vi "FrontPanelManager_Init.vi"(0 "reference in":refnum<class "FrontPanelManager.lvclass"> caption="This control should only be used when\na sub class is inheriting this class", 2 "Websocket Info":T1, 5 "error in (no error)":errorcluster) -> (14 "reference out":refnum<class "FrontPanelManager.lvclass"> caption="This indicator should only be used when\na sub class is inheriting this class", 19 "error out":errorcluster)   [LabVIEW 2014, in "FrontPanelPublisher.lvlib" / "FrontPanelManager.lvclass"]
uses:
  FrontPanelManager.lvclass
  Controls/WebsocketInfo.ctl
  WebFrontPanel_class/WebFrontPanel.lvclass
  Websocket_class/Websocket.lvclass
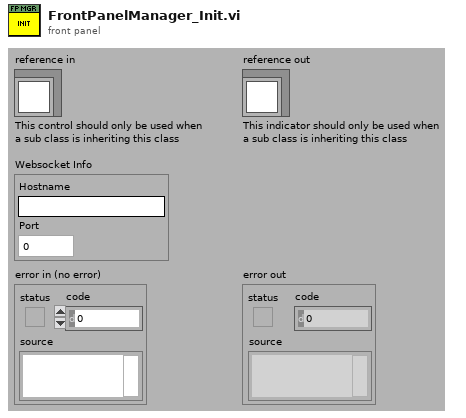
[diagram p1: front panel]
types:
  T1 = typedef "FrontPanelPublisher.lvlib/FrontPanelManager.lvclass/WebsocketInfo.ctl" = cluster{"Hostname":string, "Port":u16}
  T2 = typedef "FrontPanelPublisher.lvlib/FrontPanelManager.lvclass/ObjectAttributes.ctl" = cluster{"WebFrontPanels":refnum<class "WebFrontPanel.lvclass">[], "WFP Names":string[], "Root folder":path, "Websocket Info":T1}
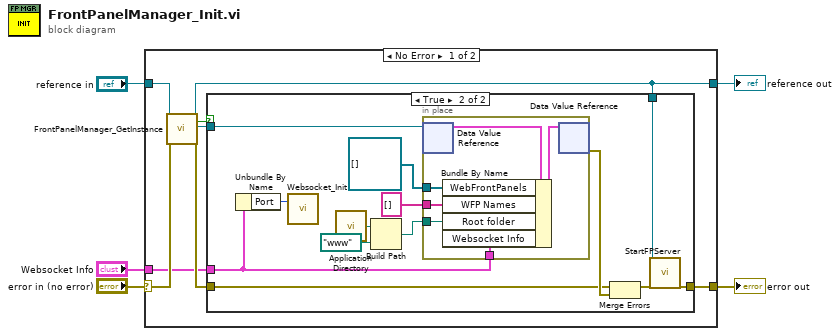
[diagram p0: block diagram]
diagram:
  n1 = case shown="No Error" "error in (no error)" {
    selector: "error in (no error)" -> [w13 w35]
    tunnel: [w6 w35] -> w4
    tunnel: "reference in" -> [w8 w34]
    tunnel: [w7 w34] -> w2
    tunnel: "Websocket Info" -> [w9 _]
    frame No Error {
      n2 = call "FrontPanelManager_GetInstance.vi"("reference in"=w8, "error in (no error)"=w13) -> ("reference out"=w7:refnum<class "FrontPanelManager.lvclass">, "NewObjectCreated"=w10:bool, "DVRRefOut"=w12:refnum<data-value>, "error out"=w11:errorcluster)  [unwired: 13 in, 1 out]
      n3 = case shown="True" w10 {
        tunnel: [w14 w16] -> w6
        tunnel: w12 -> [_ w26]
        tunnel: w11 -> [w14 w20]
        tunnel: w9 -> [_ w19]
        tunnel: w7 -> [_ w15]
        frame False {
        }
        frame True {
          n4 = Unbundle By Name(w19) -> ("Port"=w18:u16)
          n5 = call "Websocket_Init.vi"("websocket port (81)"=w18) -> ()  [unwired: 17 in, 2 out]
          n6 = call <vilib>:"Application Directory.vi"() -> ("Application Directory"=w22:path)
          n7 = Build Path(base path=w22, name or relative path=path "www") -> (appended path=w21:path)
          n8 = in-place {
            in-place-border: w21 -> [w31]
            in-place-border: string[] [] ("WFP Names") -> [w30]
            in-place-border: refnum<class "WebFrontPanel.lvclass">[] [] ("WebFrontPanels") -> [w29]
            in-place-border: w19 -> [w28]
            n9 = in-place-dvr #1(w26) -> (w32:T2)  [unwired: 1 out]
            n10 = Bundle By Name(cluster=w32, "WebFrontPanels"=w29, "WFP Names"=w30, "Root folder"=w31, "Websocket Info"=w28) -> (w33:T2)
            n11 = in-place-dvr #1(w33) -> (w27:errorcluster)  [unwired: 1 out]
          }
          n12 = Merge Errors(w20, w27) -> (w17:errorcluster)
          n13 = call "StartFPServer.vi"("reference in"=w15, "error in (no error)"=w17) -> ("error out"=w16:errorcluster)  [unwired: 16 in, 1 out]
        }
      }
    }
    frame Error {
    }
  }
  "error out" <- w4
  "reference out" <- w2
